vi "vision.vi"() -> ()   [LabVIEW 2014]
uses:
  typedefs/vision/vision enable.ctl
  typedefs/vision/vision data.ctl
panel:
  in  "Vision Data":T1
  in  "Vision Enable State":T2
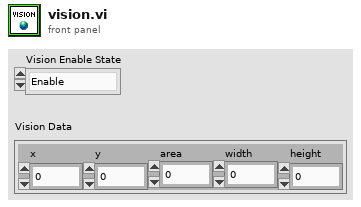
[diagram p1: front panel]
types:
  T1 = typedef "vision data.ctl" = cluster{"x":dbl, "y":dbl, "area":dbl, "width":dbl, "height":dbl}
  T2 = typedef "vision enable.ctl" = enum16{"Enable", "Disable", "Stop"}
diagram:
